vi "svx_DAQ_Facade.vi"(0 "Data In":T13, 2 "Display State In":T2={"Channel Info Array"=[], "Timing Mode"=enum."Time", "Timing Control 1"=25600.0, "Timing Control 2"=2560.0, "Timing Control 3"=16, "Timing Indicator 1"=0.1, "Reference Visible?"=FALSE, "Reference Type"=enum."<none>", "Tachometer Channel"="", "Tach Pulses Per Rev"=1, "Tach Direction"=enum."CW", "Tach Slope"=enum."Rising", "Tach Threshold"=0.0, "Trigger Channel"="", "Trigger Level"=20.0, "Pretrigger Samples"=1, "Trigger Slope"=enum."Falling", "Trigger Hysteresis"=0.0, "Logging Visible?"=FALSE, "Enable Logging"=FALSE, "Logfile Path"=path "c:/test.tdms"} caption="State" {"Timing Control 2" format="%#_6f"; "Channel Info Array"."Max" min=0.0 format="± %^#_4g"; "Channel Info Array"."Channel Type" items=["Voltage (V)"=0, "Charge (C)"=9, "-"=99, "SPL (Pa)"=3, "Force (lbf)"=6, "Force (N)"=1, "Acceleration (g) - IEPE"=2, "Acceleration (g) - Charge"=12, "Acceleration (g) - 4 wire DC Voltage"=22, "Velocity (in/s)"=7, "Velocity (mm/s)"=8, "Prox Probe (mil)"=4, "Prox Probe (mm)"=5]}, 3 "Container State":T12) -> (6 "Data Out":T13, 7 "Display State Out":T2={"Channel Info Array"=[], "Timing Mode"=enum."Time", "Timing Control 1"=25600.0, "Timing Control 2"=2560.0, "Timing Control 3"=16, "Timing Indicator 1"=0.1, "Reference Visible?"=FALSE, "Reference Type"=enum."<none>", "Tachometer Channel"="", "Tach Pulses Per Rev"=1, "Tach Direction"=enum."CW", "Tach Slope"=enum."Rising", "Tach Threshold"=0.0, "Trigger Channel"="", "Trigger Level"=20.0, "Pretrigger Samples"=1, "Trigger Slope"=enum."Falling", "Trigger Hysteresis"=0.0, "Logging Visible?"=FALSE, "Enable Logging"=FALSE, "Logfile Path"=path "c:/test.tdms"} {"Timing Control 2" format="%#_6f"; "Channel Info Array"."Max" min=0.0 format="± %^#_4g"; "Channel Info Array"."Channel Type" items=["Voltage (V)"=0, "Charge (C)"=9, "-"=99, "SPL (Pa)"=3, "Force (lbf)"=6, "Force (N)"=1, "Acceleration (g) - IEPE"=2, "Acceleration (g) - Charge"=12, "Acceleration (g) - 4 wire DC Voltage"=22, "Velocity (in/s)"=7, "Velocity (mm/s)"=8, "Prox Probe (mil)"=4, "Prox Probe (mm)"=5]}, 8 "Action":T1)   [LabVIEW 2017, in "SVX NI-DAQmx AI Configuration XControl.xctl"]
uses:
  <vilib>/addons/Sound and Vibration/svt_DAQmx/Configuration XControl/SVX NI-DAQmx AI Configuration XControl.xctl
  <vilib>/addons/Sound and Vibration/svt_DAQmx/Configuration XControl/Controls/svx_DAQ_ChannelInfo.ctl
  <vilib>/addons/Sound and Vibration/svt_DAQmx/Configuration XControl/Controls/svx_DAQ_ChannelType.ctl
  <vilib>/addons/Sound and Vibration/svt_DAQmx/Configuration XControl/Controls/svx_DAQ_Coupling.ctl
  <vilib>/addons/Sound and Vibration/svt_DAQmx/Configuration XControl/Controls/svx_DAQ_Excitation.ctl
  <vilib>/addons/Sound and Vibration/svt_DAQmx/Configuration XControl/Controls/svx_DAQ_TimingType.ctl
  <vilib>/addons/Sound and Vibration/svt_DAQmx/Configuration XControl/SubVIs/svx_DAQ_Data.ctl
  <vilib>/_xctls/Container State.ctl
  <vilib>/addons/Sound and Vibration/svt_DAQmx/Configuration XControl/SubVIs/svx_DAQ_State.ctl
  <vilib>/addons/Sound and Vibration/svt_DAQmx/Configuration XControl/Controls/svx_DAQ_ReferenceType.ctl
  <vilib>/addons/Sound and Vibration/svt_DAQmx/Configuration XControl/Controls/svx_DAQ_RotationDirection.ctl
  <vilib>/addons/Sound and Vibration/svt_DAQmx/Configuration XControl/Controls/svx_DAQ_Tach_Slope.ctl
  <vilib>/addons/Sound and Vibration/svt_DAQmx/Configuration XControl/Controls/svx_DAQ_Trigger_Slope.ctl
  <vilib>/_xctls/Action.ctl
  <vilib>/addons/Sound and Vibration/svt_DAQmx/Configuration XControl/Controls/svx_DAQ_LoadfromXMLButton.ctl
  <vilib>/addons/Sound and Vibration/svt_DAQmx/Configuration XControl/Controls/svx_DAQ_SavetoXMLButton.ctl
  <vilib>/addons/Sound and Vibration/svt_DAQmx/Configuration XControl/Controls/svx_DAQ_DetailsButton.ctl
  <vilib>/addons/Sound and Vibration/svt_DAQmx/Configuration XControl/Controls/svx_DAQ_ControlRefs.ctl
  <vilib>/_xctls/XControlSupport.lvlib
  <vilib>/Utility/miscctls.llb/LVPointTypeDef.ctl
panel:
  in  "Channel Info Array":T3[](array[typedef]) {"Max" min=0.0 format="± %^#_4g"; "Channel Type" items=["Voltage (V)"=0, "Charge (C)"=9, "-"=99, "SPL (Pa)"=3, "Force (lbf)"=6, "Force (N)"=1, "Acceleration (g) - IEPE"=2, "Acceleration (g) - Charge"=12, "Acceleration (g) - 4 wire DC Voltage"=22, "Velocity (in/s)"=7, "Velocity (mm/s)"=8, "Prox Probe (mil)"=4, "Prox Probe (mm)"=5]}
  in  "Trigger Slope":T11=enum."Rising" caption="Slope"
  in  "Tach Slope":T10 caption="Slope"
  in  "Logfile Path":path=path "c:/test.tdms"
  in  "Enable Logging":bool caption="Enable \nTDMS Logging"
  in  "Trigger Hysteresis":dbl caption="Hysteresis"
  in  "Pretrigger Samples":i32=20 caption="Pretrigger"
  in  "Trigger Level":dbl caption="Level"
  in  "Trigger Channel":string(combo)
  in  "Timing Mode":T7
  in  "Reference Type":T8
  in  "Configuration Error":T14 caption="Caption"
  in  "Save to XML":T15 caption="Caption"
  in  "Load From XML":T16 caption="Caption"
  in  "Error Picture":picture
  in  "Tachometer Channel":string(combo)
  in  "Tach Threshold":dbl caption="Threshold"
  in  "Tach Direction":T9=enum."CCW" caption="Direction"
  in  "Tach Pulses Per Rev":i32=1 caption="Pulses/Rev"
  out "Timing Indicator 1":dbl=0.1 caption="Block Duration (s)" format="%_4g"
  in  "Timing Control 3":i32=16 caption="NOT USED" min=0
  in  "Timing Control 2":dbl=2560.0 caption="Block Size" min=0.0 format="%#_6f"
  in  "Timing Control 1":dbl=25600.0 caption="Min Sample Rate (Hz)" min=0.0
  # "NI-DAQmx Channel"
  # "Channel Type (EU)"
  # "Range"
  # "Sensitivity"
  # "Excitation"
  # "Coupling"
  # "Location"
  # "Orientation"
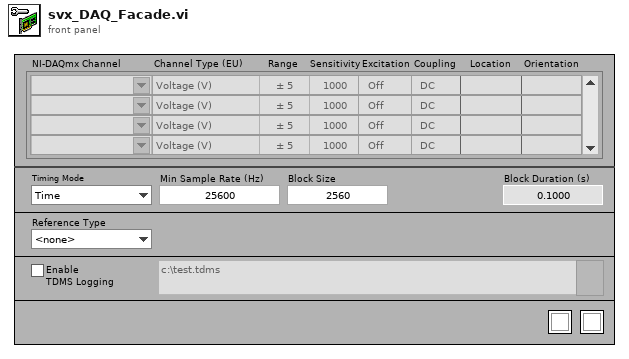
[diagram p1: front panel]
types:
  T1 = typedef "XControlSupport.lvlib/Action.ctl" = cluster{"Data Changed?":bool, "State Changed?":bool, "Action Name":string}
  T2 = typedef "SVX NI-DAQmx AI Configuration XControl.xctl/svx_DAQ_State.ctl" = cluster{"Channel Info Array":T3[], "Timing Mode":T7, "Timing Control 1":dbl, "Timing Control 2":dbl, "Timing Control 3":i32, "Timing Indicator 1":dbl, "Reference Visible?":bool, "Reference Type":T8, "Tachometer Channel":string, "Tach Pulses Per Rev":i32, "Tach Direction":T9, "Tach Slope":T10, "Tach Threshold":dbl, "Trigger Channel":string, "Trigger Level":dbl, "Pretrigger Samples":i32, "Trigger Slope":T11, "Trigger Hysteresis":dbl, "Logging Visible?":bool, "Enable Logging":bool, "Logfile Path":path}
  T3 = typedef "SVX NI-DAQmx AI Configuration XControl.xctl/svx_DAQ_ChannelInfo.ctl" = cluster{"Initialized?":bool, "DAQmx Channel":tag, "Channel Type":T4, "Max":dbl, "Sensitivity":dbl, "Excitation":bool, "Coupling":T5, "Location":string, "Orientation":string, "excitation":T6}
  T4 = typedef "SVX NI-DAQmx AI Configuration XControl.xctl/svx_DAQ_ChannelType.ctl" = u16
  T5 = typedef "SVX NI-DAQmx AI Configuration XControl.xctl/svx_DAQ_Coupling.ctl" = enum16{"AC", "DC"}
  T6 = typedef "svx_DAQ_Excitation.ctl" = enum16{"Off", "Min", "Max"}
  T7 = typedef "SVX NI-DAQmx AI Configuration XControl.xctl/svx_DAQ_TimingType.ctl" = enum16{"Time", "Frequency", "Order"}
  T8 = typedef "SVX NI-DAQmx AI Configuration XControl.xctl/svx_DAQ_ReferenceType.ctl" = enum16{"<none>", "Analog Tachometer", "Analog SW Trigger"}
  T9 = typedef "SVX NI-DAQmx AI Configuration XControl.xctl/svx_DAQ_RotationDirection.ctl" = enum16{"CW", "CCW"}
  T10 = typedef "SVX NI-DAQmx AI Configuration XControl.xctl/svx_DAQ_Tach_Slope.ctl" = enum16{"Rising", "Falling"}
  T11 = typedef "SVX NI-DAQmx AI Configuration XControl.xctl/svx_DAQ_Trigger_Slope.ctl" = enum16{"Falling", "Rising"}
  T12 = typedef "XControlSupport.lvlib/Container State.ctl" = cluster{"Indicator?":bool, "Run Mode?":bool, " Refnum":refnum<vi>}
  T13 = typedef "SVX NI-DAQmx AI Configuration XControl.xctl/svx_DAQ_Data.ctl" = refnum<k21>
  T14 = typedef "SVX NI-DAQmx AI Configuration XControl.xctl/svx_DAQ_DetailsButton.ctl" = bool
  T15 = typedef "SVX NI-DAQmx AI Configuration XControl.xctl/svx_DAQ_SavetoXMLButton.ctl" = bool
  T16 = typedef "SVX NI-DAQmx AI Configuration XControl.xctl/svx_DAQ_LoadfromXMLButton.ctl" = bool
  T17 = typedef "SVX NI-DAQmx AI Configuration XControl.xctl/svx_DAQ_ControlRefs.ctl" = cluster{"Channel Info Array":refnum<vi>, "Timing Mode":refnum<vi>, "Timing Control 1":refnum<vi>, "Timing Control 2":refnum<vi>, "Timing Control 3":refnum<vi>, "Timing Indicator 1":refnum<vi>, "Reference Type":refnum<vi>, "Tachometer Channel":refnum<vi>, "Tach Pulses Per Rev":refnum<vi>, "Tach Direction":refnum<vi>, "Tach Slope":refnum<vi>, "Tach Threshold":refnum<vi>, "Error Picture":refnum<vi>, "Configuration Error":refnum<vi>, "Load From XML":refnum<vi>, "Save to XML":refnum<vi>, "Trigger Channel":refnum<vi>, "Trigger Level":refnum<vi>, "Trigger Slope":refnum<vi>, "Pretrigger Samples":refnum<vi>, "Trigger Hysteresis":refnum<vi>, "Enable Logging":refnum<vi>, "Logfile Path":refnum<vi>, "Task Configuration":refnum<vi>, "Splitter":refnum<vi>}
  T18 = enum8{"Enabled", "Disabled", "Disabled and Grayed Out"}
  T19 = typedef "LVPointTypeDef.ctl" = cluster{"Horizontal":i16, "Vertical":i16}
  T20 = typedef "LVRectTypeDef.ctl" = cluster{"Left":i16, "Top":i16, "Right":i16, "Bottom":i16}
  T21 = typedef "eventvkey.ctl" = enum16{"ASCII", "Enter", "Return", "Shift", "Ctrl", "Alt", "Cmd", "Opt", "Caps", "NumLock", "Clear", "Break", "Up", "Down", "Left", "Right", "Insert", "Delete", "Home", "End", "PageUp", "PageDown", "Escape", "Help", "Pause", "ScrollLock", "F1", "F2", "F3", "F4", "F5", "F6", "F7", "F8", "F9", "F10", "F11", "F12", "F13", "F14", "F15", "F16", "F17", "F18", "F19", "F20", "F21", "F22", "F23", "F24", "Play", "VolumeUp", "VolumeDown", "Mute", "Two Byte Char"}
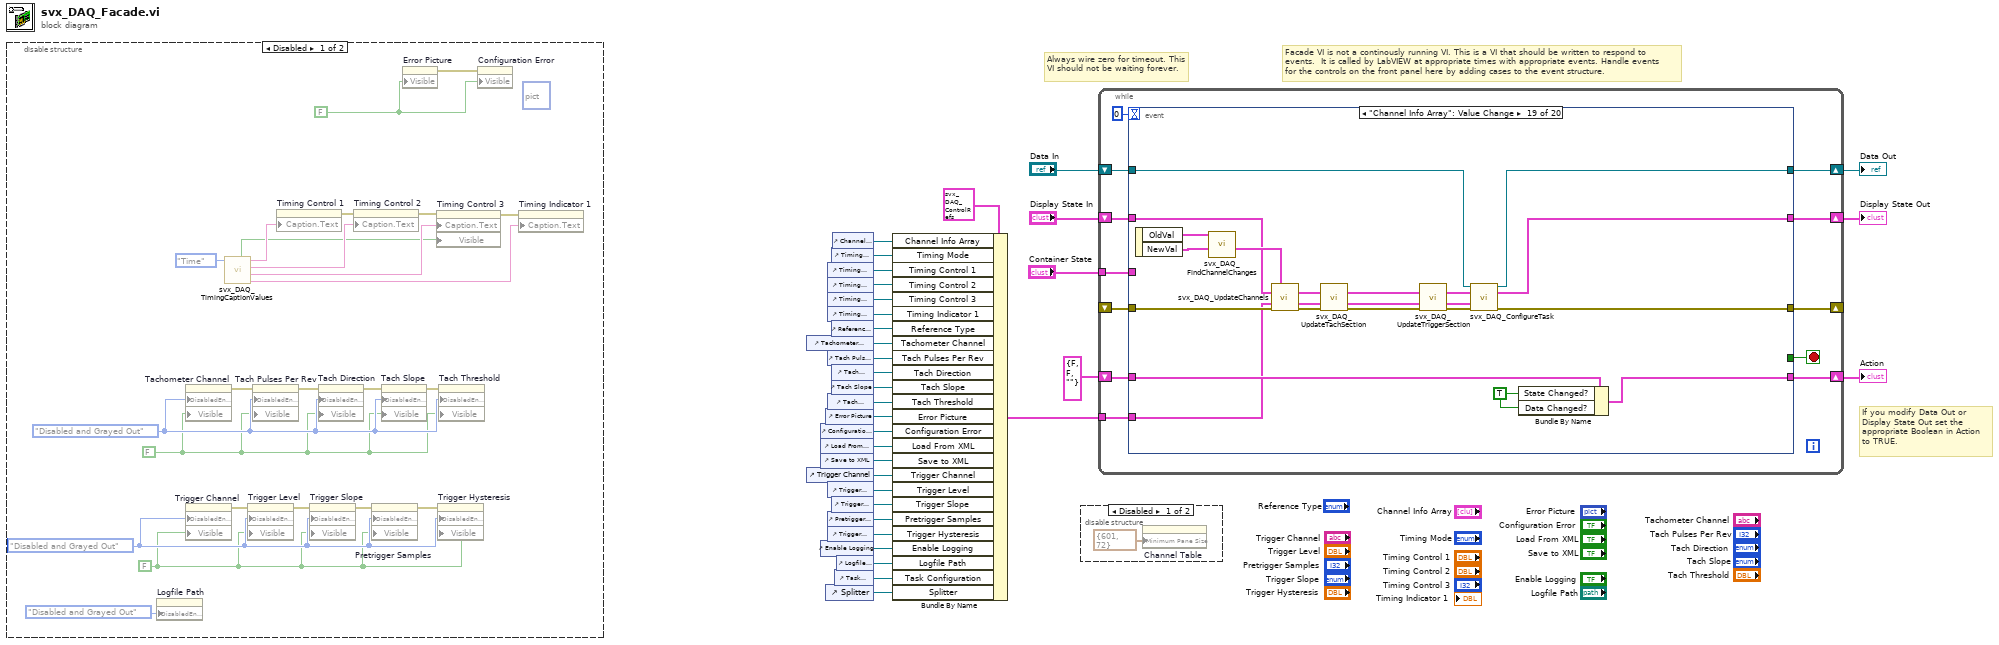
[diagram p0: block diagram]
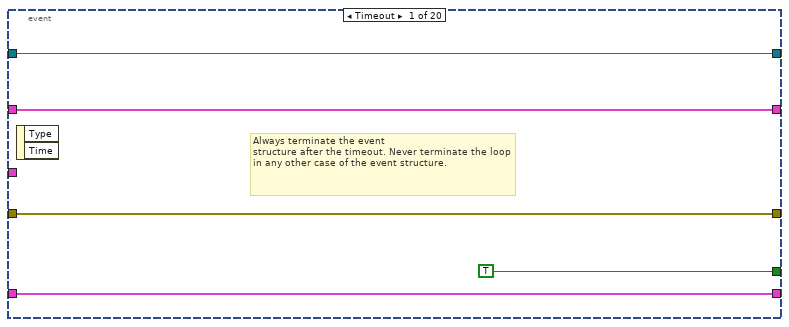
[diagram p4: hidden frame]
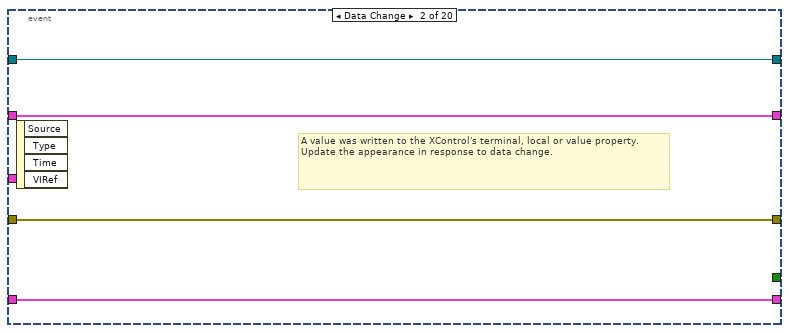
[diagram p5: hidden frame]
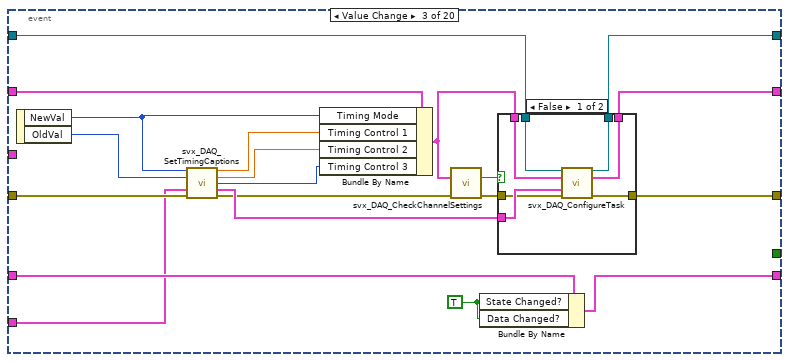
[diagram p6: hidden frame]
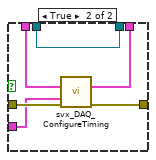
[diagram p7: hidden frame]
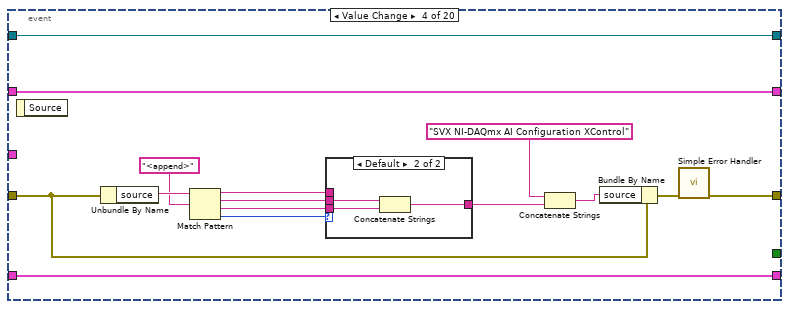
[diagram p8: hidden frame]
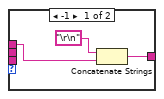
[diagram p9: hidden frame]
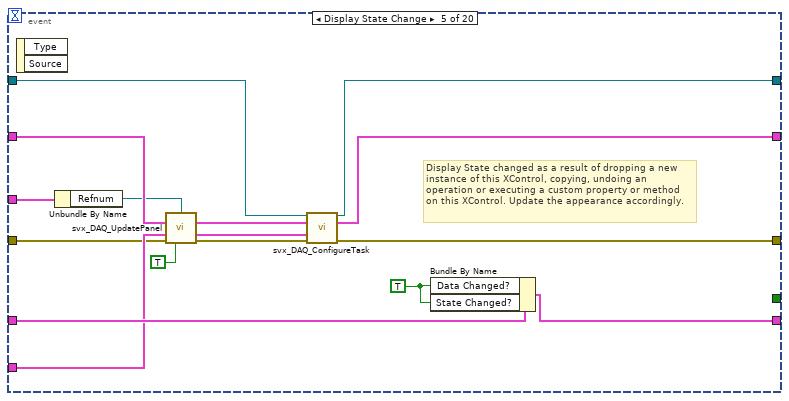
[diagram p10: hidden frame]
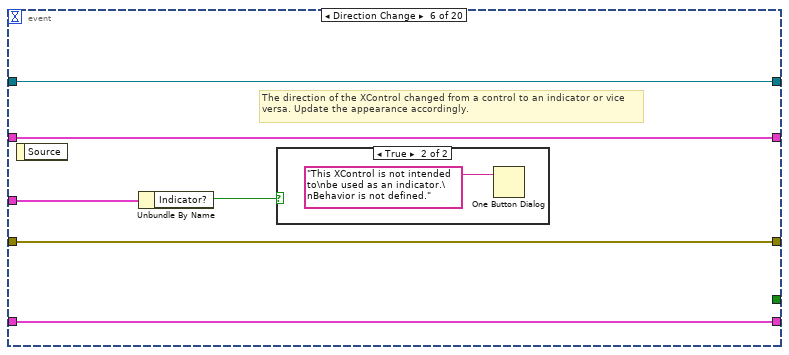
[diagram p11: hidden frame]
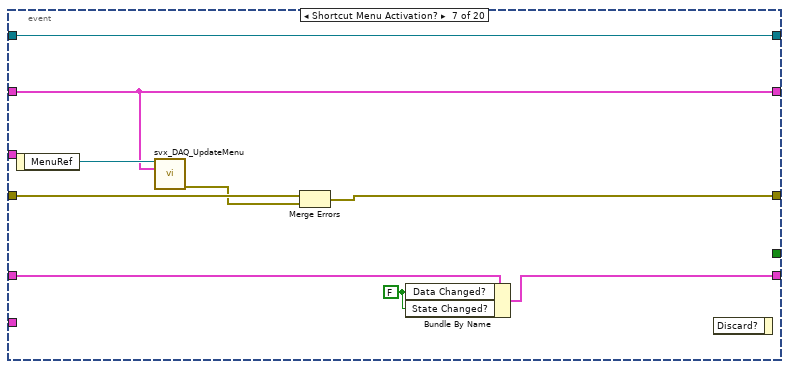
[diagram p13: hidden frame]
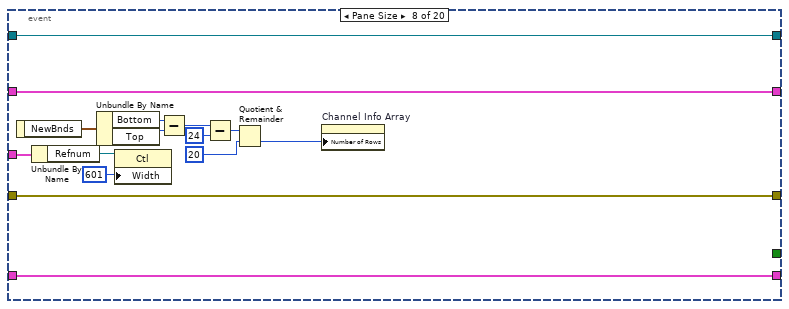
[diagram p14: hidden frame]
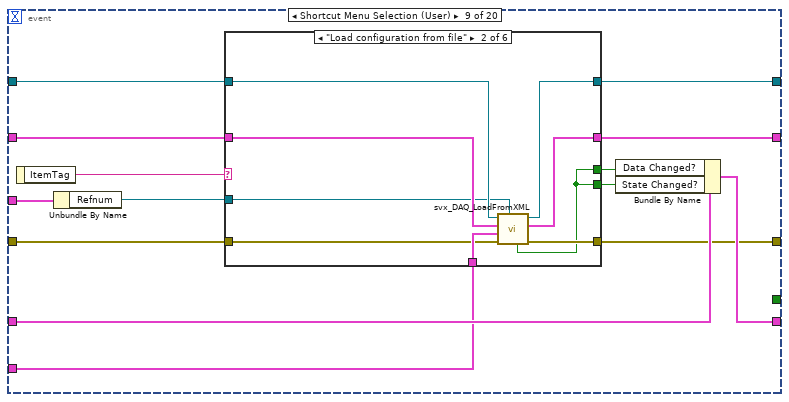
[diagram p15: hidden frame]
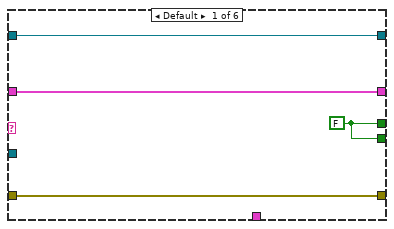
[diagram p16: hidden frame]
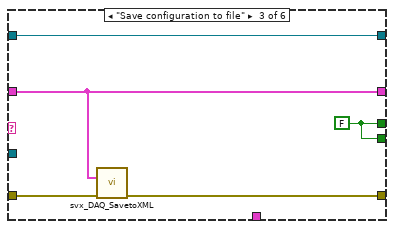
[diagram p17: hidden frame]
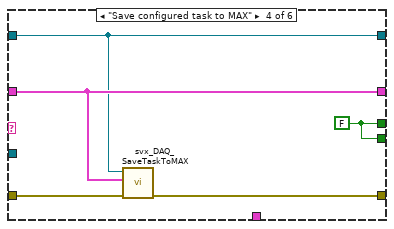
[diagram p18: hidden frame]
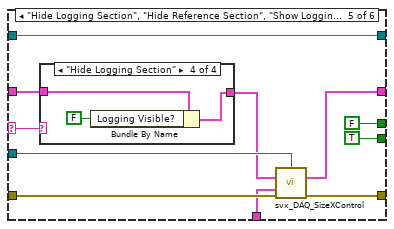
[diagram p19: hidden frame]
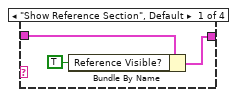
[diagram p20: hidden frame]
diagram:
  # "Facade VI is not a continously running VI. This is a VI that should be written to respond to events.  It is called by LabVIEW at appropriate times with appropriate events. Handle events for the controls on the front panel here by adding cases to the event structure."
  # "Always wire zero for timeout. This\nVI should not be waiting forever."
  # "If you modify Data Out or\nDisplay State Out set the\nappropriate Boolean in Action\nto TRUE."
  n1 = disable-structure shown="Disabled" {
    frame Disabled {
      w38 = FALSE ("Visible")
      w39 = T18."Disabled and Grayed Out" ("Disabled")
      w40 = FALSE ("Visible")
      w41 = T18."Disabled and Grayed Out" ("Disabled")
      (unwired) picture bytes[2913] ("Error Picture")
      w55 = FALSE ("Visible")
      n2 = property on="Logfile Path" class="Path"("DisabledEnum"=T18."Disabled and Grayed Out" ("Disabled")) -> ()  [unwired: 2 in, 2 out]
      n3 = property on="Tachometer Channel" class="CmbBox"("DisabledEnum"=w41, "Visible"=w40) -> (error out=w47:errorcluster)  [unwired: 2 in, 1 out]
      n4 = property on="Trigger Channel" class="CmbBox"("DisabledEnum"=w39, "Visible"=w38) -> (error out=w45:errorcluster)  [unwired: 2 in, 1 out]
      n5 = call <vilib>:"svx_DAQ_TimingCaptionValues.vi"("Timing Mode"=svx_DAQ_TimingType."Time") -> ("Timing Indicator 1 Caption"=w50:string, "Timing Control 3 Caption"=w51:string, "Timing Control 2 Caption"=w57:string, "Timing Control 1 Caption"=w58:string, "Timing Control 3 Visible?"=w49:bool)  [unwired: 6 in]
      n6 = property on="Trigger Level" class="DigNum (strict)"(error in=w45, "DisabledEnum"=w39, "Visible"=w38) -> (error out=w37:errorcluster)  [unwired: 1 in, 1 out]
      n7 = property on="Tach Pulses Per Rev" class="DigNum (strict)"(error in=w47, "DisabledEnum"=w41, "Visible"=w40) -> (error out=w48:errorcluster)  [unwired: 1 in, 1 out]
      n8 = property on="Timing Control 1" class="DigNum (strict)"("Caption.Text"=w58) -> (error out=w56:errorcluster)  [unwired: 2 in, 1 out]
      n9 = property on="Trigger Slope" class="Enum (strict)"(error in=w37, "DisabledEnum"=w39, "Visible"=w38) -> (error out=w36:errorcluster)  [unwired: 1 in, 1 out]
      n10 = property on="Tach Direction" class="Enum (strict)"(error in=w48, "DisabledEnum"=w41, "Visible"=w40) -> (error out=w43:errorcluster)  [unwired: 1 in, 1 out]
      n11 = property on="Timing Control 2" class="DigNum (strict)"(error in=w56, "Caption.Text"=w57) -> (error out=w53:errorcluster)  [unwired: 1 in, 1 out]
      n12 = property on="Pretrigger Samples" class="DigNum (strict)"(error in=w36, "DisabledEnum"=w39, "Visible"=w38) -> (error out=w46:errorcluster)  [unwired: 1 in, 1 out]
      n13 = property on="Tach Slope" class="Enum (strict)"(error in=w43, "DisabledEnum"=w41, "Visible"=w40) -> (error out=w42:errorcluster)  [unwired: 1 in, 1 out]
      n14 = property on="Error Picture" class="Pict"("Visible"=w55) -> (error out=w54:errorcluster)  [unwired: 2 in, 1 out]
      n15 = property on="Timing Control 3" class="DigNum (strict)"(error in=w53, "Caption.Text"=w51, "Visible"=w49) -> (error out=w52:errorcluster)  [unwired: 1 in, 1 out]
      n16 = property on="Trigger Hysteresis" class="DigNum (strict)"(error in=w46, "DisabledEnum"=w39, "Visible"=w38) -> ()  [unwired: 1 in, 2 out]
      n17 = property on="Tach Threshold" class="DigNum (strict)"(error in=w42, "DisabledEnum"=w41, "Visible"=w40) -> ()  [unwired: 1 in, 2 out]
      n18 = property on="Configuration Error" class="Bool"(error in=w54, "Visible"=w55) -> ()  [unwired: 1 in, 2 out]
      n19 = property on="Timing Indicator 1" class="DigNum (strict)"(error in=w52, "Caption.Text"=w50) -> ()  [unwired: 1 in, 2 out]
    }
    frame Enabled {
    }
  }
  n20 = control-ref of="Tachometer Channel"() -> (w24:refnum<vi>)
  n21 = control-ref of="Trigger Channel"() -> (w13:refnum<vi>)
  n22 = control-ref of="Configuration Error"() -> (w19:refnum<vi>)
  n23 = control-ref of="Load From XML"() -> (w18:refnum<vi>)
  n24 = control-ref of="Save to XML"() -> (w17:refnum<vi>)
  n25 = control-ref of="Enable Logging"() -> (w8:refnum<vi>)
  n26 = control-ref of="Error Picture"() -> (w20:refnum<vi>)
  n27 = control-ref of="Splitter"() -> (w3:refnum<vi>)
  n28 = control-ref of="Timing Control 1"() -> (w27:refnum<vi>)
  n29 = control-ref of="Timing Control 2"() -> (w26:refnum<vi>)
  n30 = control-ref of="Timing Control 3"() -> (w16:refnum<vi>)
  n31 = control-ref of="Timing Indicator 1"() -> (w25:refnum<vi>)
  n32 = control-ref of="Tach Pulses Per Rev"() -> (w23:refnum<vi>)
  n33 = control-ref of="Tach Threshold"() -> (w21:refnum<vi>)
  n34 = control-ref of="Trigger Level"() -> (w12:refnum<vi>)
  n35 = control-ref of="Pretrigger Samples"() -> (w11:refnum<vi>)
  n36 = control-ref of="Trigger Hysteresis"() -> (w10:refnum<vi>)
  n37 = control-ref of="Timing Mode"() -> (w14:refnum<vi>)
  n38 = control-ref of="Reference Type"() -> (w9:refnum<vi>)
  n39 = control-ref of="Tach Direction"() -> (w22:refnum<vi>)
  n40 = control-ref of="Tach Slope"() -> (w6:refnum<vi>)
  n41 = control-ref of="Trigger Slope"() -> (w5:refnum<vi>)
  n42 = control-ref of="Channel Info Array"() -> (w1:refnum<vi>)
  n43 = control-ref of="Task Configuration"() -> (w4:refnum<vi>)
  n44 = control-ref of="Logfile Path"() -> (w7:refnum<vi>)
  n45 = Bundle By Name(cluster=T17 {"Channel Info Array"=refnum, "Timing Mode"=refnum, "Timing Control 1"=refnum, "Timing Control 2"=refnum, "Timing Control 3"=refnum, "Timing Indicator 1"=refnum, "Reference Type"=refnum, "Tachometer Channel"=refnum, "Tach Pulses Per Rev"=refnum, "Tach Direction"=refnum, "Tach Slope"=refnum, "Tach Threshold"=refnum, "Error Picture"=refnum, "Configuration Error"=refnum, "Load From XML"=refnum, "Save to XML"=refnum, "Trigger Channel"=refnum, "Trigger Level"=refnum, "Trigger Slope"=refnum, "Pretrigger Samples"=refnum, "Trigger Hysteresis"=refnum, "Enable Logging"=refnum, "Logfile Path"=refnum, "Task Configuration"=refnum, "Splitter"=refnum}, "Channel Info Array"=w1, "Timing Mode"=w14, "Timing Control 1"=w27, "Timing Control 2"=w26, "Timing Control 3"=w16, "Timing Indicator 1"=w25, "Reference Type"=w9, "Tachometer Channel"=w24, "Tach Pulses Per Rev"=w23, "Tach Direction"=w22, "Tach Slope"=w6, "Tach Threshold"=w21, "Error Picture"=w20, "Configuration Error"=w19, "Load From XML"=w18, "Save to XML"=w17, "Trigger Channel"=w13, "Trigger Level"=w12, "Trigger Slope"=w5, "Pretrigger Samples"=w11, "Trigger Hysteresis"=w10, "Enable Logging"=w8, "Logfile Path"=w7, "Task Configuration"=w4, "Splitter"=w3) -> (w29:T17)
  n46 = disable-structure shown="Disabled" {
    frame Disabled {
      n47 = property on="Channel Table" class="Pane"("Minimum Pane Size"=T19 {"Horizontal"=601, "Vertical"=72}) -> ()  [unwired: 2 in, 2 out]
    }
    frame Enabled {
    }
  }
  n48 = while {
    shift-right: [w70] -> w32
    shift-left: "Display State In" -> [w71]
    tunnel: "Container State" -> [w67]
    shift-right: [w60] -> w28
    shift-left: "Data In" -> [w66]
    shift-right: [w64] -> w31
    shift-left: T1 {"Data Changed?"=FALSE, "State Changed?"=FALSE, "Action Name"=""} ("Action") -> [w65]
    tunnel: w29 -> [w63]
    shift-right: [w62] -> _
    shift-left: _ -> [w61]
    stop <- w69 stop-if-true
    n49 = event shown="[18] \"Channel Info Array\": Value Change" {
      selector: _ -> [_ _ _ _ _ _ _ _ _ _ _ _ _ _ _ _ _ _ _ _]
      dyn-events: _ -> [_ _ _ _ _ _ _ _ _ _ _ _ _ _ _ _ _ _ _ _]
      timeout: 0 -> [_ _ _ _ _ _ _ _ _ _ _ _ _ _ _ _ _ _ _ _]
      tunnel: w71 -> [w74 w79 w97 w128 w143 w155 w164 w180 w195 w268 w301 w309 w316 w334 w360 w398 w440 w461 w510 w530]
      tunnel: [w74 w79 w92 w128 w145 w155 w164 w180 w188 w267 w291 w310 w316 w331 w357 w402 w443 w458 w511 w530] -> w70
      tunnel: [TRUE _ _ _ _ _ _ _ _ _ _ _ _ _ _ _ _ _ _ _] -> w69
      tunnel: w67 -> [_ _ _ _ w137 w156 _ w169 w184 w272 _ w305 _ _ _ _ _ _ _ _]
      tunnel: w66 -> [w72 w78 w85 w126 w150 w153 w166 w181 w187 w266 w293 w311 w317 w330 w359 w404 w445 w460 w513 w535]
      tunnel: [w72 w78 w96 w126 w149 w153 w166 w181 w189 w263 w292 w313 w317 w329 w358 w403 w444 w459 w518 w535] -> w60
      tunnel: [w75 w80 w99 w127 w147 w154 w161 w178 w193 w264 w299 w302 w318 w335 w361 w405 w446 w463 w520 w529] -> w64
      tunnel: w65 -> [w75 w80 w100 w127 w148 w154 w163 w178 w194 w265 w300 w303 w318 w336 w362 w406 w447 w464 w519 w529]
      tunnel: w63 -> [_ _ w91 _ w142 _ _ _ w186 w269 w296 w312 _ w321 w353 w395 w438 w453 w515 _]
      tunnel: [w73 w77 w94 w125 w144 w152 w158 w179 w190 w270 w295 w308 w314 w332 w356 w401 w442 w457 w512 w532] -> w62
      tunnel: w61 -> [w73 w77 w93 w121 w141 w152 w160 w179 w192 w271 w297 w307 w315 w325 w355 w396 w436 w454 w516 w532]
      event Timeout {
        # "Always terminate the event\nstructure after the timeout. Never terminate the loop in any other case of the event structure."
        n50 = event-data() -> ()  [unwired: 1 in, 2 out]
      }
      event Data Change {
        # "A value was written to the XControl's terminal, local or value property.\nUpdate the appearance in response to data change."
        n51 = event-data() -> ()  [unwired: 1 in, 4 out]
      }
      event Value Change {
        w95 = TRUE ("State Changed?")
        n52 = event-data() -> ("NewVal"=w98:T7, "OldVal"=w89:T7)  [unwired: 1 in]
        n53 = call <vilib>:"svx_DAQ_SetTimingCaptions.vi"("Timing Mode (new)"=w98, "Timing Mode (old)"=w89, "Reference Cluster"=w91, "error in (no error)"=w93) -> ("Timing Control 1"=w88:dbl, "Timing Control 2"=w87:dbl, "Timing Control 3"=w86:i32, "Reference Cluster Out"=w90:T17, "error out"=w83:errorcluster)  [unwired: 7 in]
        n54 = Bundle By Name(cluster=w97, "Timing Mode"=w98, "Timing Control 1"=w88, "Timing Control 2"=w87, "Timing Control 3"=w86) -> (w84:T2)
        n55 = call <vilib>:"svx_DAQ_CheckChannelSettings.vi"("Display State In"=w84, "error in (no error)"=w83) -> ("Empty Channel List?"=w81:bool, "error out"=w82:errorcluster)  [unwired: 9 in, 3 out]
        n56 = Bundle By Name(cluster=w100, "State Changed?"=w95, "Data Changed?"=w95) -> (w99:T1)
        n57 = case shown="False" w81 {
          tunnel: [w107 w108] -> w96
          tunnel: [w106 w112] -> w94
          tunnel: [w105 w110] -> w92
          tunnel: w90 -> [w104 w109]
          tunnel: w85 -> [w103 w108]
          tunnel: w84 -> [w102 w111]
          tunnel: w82 -> [w101 w113]
          frame False {
            n58 = call <vilib>:"svx_DAQ_ConfigureTask.vi"("Task In"=w103, "Display State In"=w102, "cluster"=w104, "error in"=w101) -> ("task out"=w107:refnum<k21>, "Display State Out"=w105:T2, "error out"=w106:errorcluster)  [unwired: 8 in, 1 out]
          }
          frame True {
            n59 = call <vilib>:"svx_DAQ_ConfigureTiming.vi"("Display State In"=w111, "cluster"=w109, "Error In (no error)"=w113) -> ("Display State Out"=w110:T2, "error out"=w112:errorcluster)  [unwired: 9 in, 2 out]
          }
        }
      }
      event Value Change {
        n60 = event-data() -> ()  [unwired: 1 in, 1 out]
        n61 = Unbundle By Name(w121) -> ("source"=w124:string)
        n62 = Match Pattern(string=w124, regular expression="<append>") -> (before substring=w117:string, match substring=w116:string, after substring=w115:string, offset past match=w119:i32)  [unwired: 1 in]
        n63 = case shown="Default" w119 {
          tunnel: [w129 w132] -> w118
          tunnel: w117 -> [w130 _]
          tunnel: w116 -> [_ w134]
          tunnel: w115 -> [_ w133]
          frame -1 {
            n64 = Concatenate Strings("\r\n", w130) -> (w129:string)
          }
          frame Default {
            n65 = Concatenate Strings(w134, w133) -> (w132:string)
          }
        }
        n66 = Concatenate Strings("SVX NI-DAQmx AI Configuration XControl" ("error source (\" \")"), w118) -> (w114:string)
        n67 = Bundle By Name(cluster=w121, "source"=w114) -> (w120:errorcluster)
        n68 = call <vilib>:"Simple Error Handler.vi"("error in (no error)"=w120) -> ("error out"=w125:errorcluster)  [unwired: 4 in, 4 out]
      }
      event Display State Change {
        w146 = TRUE ("Data Changed?")
        # "Display State changed as a result of dropping a new instance of this XControl, copying, undoing an operation or executing a custom property or method on this XControl. Update the appearance accordingly."
        n69 = event-data() -> ()  [unwired: 1 in, 2 out]
        n70 = Unbundle By Name(w137) -> ("Refnum"=w136:refnum<vi>)
        n71 = call <vilib>:"svx_DAQ_UpdatePanel.vi"("XControl Ref"=w136, "State"=w143, "cluster"=w142, "error in (no error)"=w141, "display state change"=TRUE) -> ("State Out"=w138:T2, "cluster"=w139:T17, "error out"=w140:errorcluster)  [unwired: 8 in]
        n72 = call <vilib>:"svx_DAQ_ConfigureTask.vi"("Task In"=w150, "Display State In"=w138, "cluster"=w139, "error in"=w140) -> ("task out"=w149:refnum<k21>, "Display State Out"=w145:T2, "error out"=w144:errorcluster)  [unwired: 8 in, 1 out]
        n73 = Bundle By Name(cluster=w148, "Data Changed?"=w146, "State Changed?"=w146) -> (w147:T1)
      }
      event Direction Change {
        # "The direction of the XControl changed from a control to an indicator or vice versa. Update the appearance accordingly."
        n74 = event-data() -> ()  [unwired: 1 in, 1 out]
        n75 = Unbundle By Name(w156) -> ("Indicator?"=w151:bool)
        n76 = case shown="True" w151 {
          frame False {
          }
          frame True {
            n77 = One Button Dialog(message="This XControl is not intended to\nbe used as an indicator.\nBehavior is not defined.") -> ()  [unwired: 1 in, 1 out]
          }
        }
      }
      event Shortcut Menu Activation? {
        w162 = FALSE ("Data Changed?")
        n78 = event-data() -> ("MenuRef"=w165:refnum<k9>)  [unwired: 1 in]
        n79 = call <vilib>:"svx_DAQ_UpdateMenu.vi"("MenuRef"=w165, "Display State In"=w164) -> ("error out"=w159:errorcluster)  [unwired: 13 in]
        n80 = Merge Errors(w160, w159) -> (w158:errorcluster)
        n81 = Bundle By Name(cluster=w163, "Data Changed?"=w162, "State Changed?"=w162) -> (w161:T1)
        n82 = event-data() -> ()  [unwired: 2 in, 1 out]
      }
      event Pane Size {
        n83 = event-data() -> ("NewBnds"=w177:T20)  [unwired: 1 in]
        n84 = Unbundle By Name(w169) -> ("Refnum"=w168:refnum<vi>)
        n85 = Unbundle By Name(w177) -> ("Bottom"=w175:i16, "Top"=w176:i16)
        n86 = property class="Ctl"(reference=w168, "Width"=u32 601 ("XControl:Container Bounds:Width")) -> ()  [unwired: 1 in, 2 out]
        n87 = Subtract(x=w175, y=w176) -> (x-y=w174:i16)
        n88 = Subtract(x=w174, y=i16 24) -> (x-y=w172:i16)
        n89 = Quotient & Remainder(x=w172, y=i16 20) -> (floor(x/y)=w170:i16)  [unwired: 1 out]
        n90 = property on="Channel Info Array" class="Arr (strict)"("Number of Rows"=w170) -> ()  [unwired: 2 in, 2 out]
      }
      event Shortcut Menu Selection (User) {
        n91 = event-data() -> ("ItemTag"=w191:string)  [unwired: 1 in]
        n92 = Unbundle By Name(w184) -> ("Refnum"=w183:refnum<vi>)
        n93 = case shown="\"Load configuration from file\"" w191 {
          selector: w191 -> [_ _ _ _ w219 _]
          tunnel: w195 -> [w199 w205 w212 w216 w221 w251]
          tunnel: [w199 w206 w212 w216 w223 w244] -> w188
          tunnel: w192 -> [w198 w202 w211 w218 w226 w247]
          tunnel: [w198 w203 w210 w217 w222 w249] -> w190
          tunnel: [w197 w207 w213 w215 w227 w252] -> w189
          tunnel: w187 -> [w197 w208 w213 w215 w227 w252]
          tunnel: w186 -> [_ w204 _ _ w225 w243]
          tunnel: [w196 w201 w209 w214 FALSE ("State and Data Changed?") FALSE ("State and Data Changed?")] -> w185
          tunnel: w183 -> [_ w200 _ _ w224 w248]
          tunnel: [w196 w201 w209 w214 TRUE ("State and Data Changed?") w242] -> w182
          frame Default {
            w196 = FALSE ("State and Data Changed?")
          }
          frame "Load configuration from file" {
            n94 = call <vilib>:"svx_DAQ_LoadFromXML.vi"("XControl Ref"=w200, "error in (no error)"=w202, "cluster"=w204, "Display State In"=w205, "Data In"=w208) -> ("error out"=w203:errorcluster, "Display State Out"=w206:T2, "Data Out"=w207:T13, "State and Data Changed?"=w201:bool)  [unwired: 3 in]
          }
          frame "Save configuration to file" {
            w209 = FALSE ("State and Data Changed?")
            n95 = call <vilib>:"svx_DAQ_SavetoXML.vi"("State"=w212, "error in (no error)"=w211) -> ("error out"=w210:errorcluster)  [unwired: 12 in, 1 out]
          }
          frame "Save configured task to MAX" {
            w214 = FALSE ("State and Data Changed?")
            n96 = call <vilib>:"svx_DAQ_SaveTaskToMAX.vi"("error in (no error)"=w218, "Display State In"=w216, "Task In"=w215) -> ("error out"=w217:errorcluster)  [unwired: 8 in]
          }
          frame "Hide Logging Section", "Hide Reference Section", "Show Logging Section", "Show Reference Section" {
            n97 = case shown="\"Hide Logging Section\"" w219 {
              tunnel: w221 -> [w231 w234 w237 w240]
              tunnel: [w230 w233 w236 w239] -> w220
              frame "Show Reference Section", Default {
                n98 = Bundle By Name(cluster=w231, "Reference Visible?"=TRUE) -> (w230:T2)
              }
              frame "Hide Reference Section" {
                n99 = Bundle By Name(cluster=w234, "Reference Visible?"=FALSE) -> (w233:T2)
              }
              frame "Show Logging Section" {
                n100 = Bundle By Name(cluster=w237, "Logging Visible?"=TRUE ("Reference Visible?")) -> (w236:T2)
              }
              frame "Hide Logging Section" {
                n101 = Bundle By Name(cluster=w240, "Logging Visible?"=FALSE ("Reference Visible?")) -> (w239:T2)
              }
            }
            n102 = call <vilib>:"svx_DAQ_SizeXControl.vi"("XControl Ref"=w224, "State"=w220, "Reference Cluster"=w225, "error in (no error)"=w226) -> ("State Out"=w223:T2, "error out"=w222:errorcluster)  [unwired: 9 in, 1 out]
          }
          frame "Unflatten Channel List" {
            n103 = call <vilib>:"svx_DAQ_ExplodeChannels.vi"("Display State In"=w251, "error in (no error)"=w247) -> ("Display State Out"=w245:T2, "State Updated?"=w242:bool, "error out"=w246:errorcluster)  [unwired: 11 in]
            n104 = case shown="True" w242 {
              tunnel: [w253 w260] -> w249
              tunnel: w248 -> [_ w259]
              tunnel: w246 -> [w253 w258]
              tunnel: w245 -> [w254 w257]
              tunnel: [w254 w256] -> w244
              tunnel: w243 -> [_ w255]
              frame False {
              }
              frame True {
                n105 = call <vilib>:"svx_DAQ_UpdatePanel.vi"("XControl Ref"=w259, "State"=w257, "cluster"=w255, "error in (no error)"=w258) -> ("State Out"=w256:T2, "error out"=w260:errorcluster)  [unwired: 9 in, 1 out]
              }
            }
          }
        }
        n106 = Bundle By Name(cluster=w194, "Data Changed?"=w185, "State Changed?"=w182) -> (w193:T1)
      }
      event Exec State Change {
        # "The VI owning the XControl changed from Edit Mode  to Run Mode or vice versa.\nUpdate the appearance accordingly."
        # "Handle Edit Mode & Run Mode\ncase differently"
        n107 = event-data() -> ()  [unwired: 1 in, 1 out]
        n108 = Unbundle By Name(w272) -> ("Run Mode?"=w261:bool)
        n109 = case shown="False" w261 {
          tunnel: w271 -> [w279 w280]
          tunnel: [w278 w280] -> w270
          tunnel: w269 -> [w277 _]
          tunnel: w268 -> [w276 w282]
          tunnel: [w275 w282] -> w267
          tunnel: [w274 w281] -> w263
          tunnel: w266 -> [w273 w281]
          frame False {
            n110 = call <vilib>:"svx_DAQ_ConfigureTask.vi"("Task In"=w273, "Display State In"=w276, "cluster"=w277, "error in"=w279) -> ("task out"=w274:refnum<k21>, "Display State Out"=w275:T2, "error out"=w278:errorcluster)  [unwired: 8 in, 1 out]
          }
          frame True {
          }
        }
        n111 = Not(x=w261) -> (.not. x?=w262:bool)
        n112 = Bundle By Name(cluster=w265, "Data Changed?"=w262) -> (w264:T1)
      }
      event Value Change {
        n113 = event-data() -> ("NewVal"=w289:T8)  [unwired: 1 in]
        n114 = Bundle By Name(cluster=w301, "Reference Type"=w289) -> (w290:T2)
        n115 = call <vilib>:"svx_DAQ_UpdateTachSection.vi"("State"=w290, "cluster"=w296, "error in (no error)"=w297) -> ("State Out"=w284:T2, "cluster"=w286:T17, "error out"=w288:errorcluster)  [unwired: 10 in]
        n116 = call <vilib>:"svx_DAQ_UpdateTriggerSection.vi"("State"=w284, "Reference Cluster"=w286, "error in (no error)"=w288) -> ("State Out"=w283:T2, "Reference Cluster Out"=w285:T17, "error out"=w287:errorcluster)  [unwired: 10 in]
        n117 = call <vilib>:"svx_DAQ_ConfigureTask.vi"("Task In"=w293, "Display State In"=w283, "cluster"=w285, "error in"=w287) -> ("task out"=w292:refnum<k21>, "Display State Out"=w291:T2, "error out"=w295:errorcluster)  [unwired: 8 in, 1 out]
        n118 = Bundle By Name(cluster=w300, "State Changed?"=TRUE, "Data Changed?"=TRUE ("State Changed?")) -> (w299:T1)
      }
      event Value Change {
        n119 = event-data() -> ()  [unwired: 1 in, 1 out]
        n120 = Unbundle By Name(w305) -> ("Refnum"=w304:refnum<vi>)
        n121 = call <vilib>:"svx_DAQ_LoadFromXML.vi"("XControl Ref"=w304, "error in (no error)"=w307, "cluster"=w312, "Display State In"=w309, "Data In"=w311) -> ("error out"=w308:errorcluster, "Display State Out"=w310:T2, "Data Out"=w313:T13, "State and Data Changed?"=w306:bool)  [unwired: 3 in]
        n122 = Bundle By Name(cluster=w303, "State Changed?"=w306, "Data Changed?"=w306) -> (w302:T1)
      }
      event Value Change {
        n123 = event-data() -> ()  [unwired: 1 in, 1 out]
        n124 = call <vilib>:"svx_DAQ_SavetoXML.vi"("State"=w316, "error in (no error)"=w315) -> ("error out"=w314:errorcluster)  [unwired: 12 in, 1 out]
      }
      event "Enable Logging": Value Change {
        n125 = event-data() -> ("NewVal"=w333:bool)  [unwired: 1 in]
        n126 = Bundle By Name(cluster=w334, "Enable Logging"=w333) -> (w323:T2)
        n127 = call <vilib>:"svx_DAQ_UpdateLogSection.vi"("State"=w323, "Reference Cluster"=w321, "error in (no error)"=w325) -> ("State Out"=w322:T2, "error out"=w324:errorcluster)  [unwired: 10 in, 1 out]
        n128 = call <vilib>:"svx_DAQ_CheckChannelSettings.vi"("Display State In"=w322, "error in (no error)"=w324) -> ("Empty Channel List?"=w320:bool, "error out"=w328:errorcluster)  [unwired: 9 in, 3 out]
        n129 = Not(x=w320) -> (.not. x?=w319:bool)
        n130 = case shown="True" w319 {
          tunnel: [w338 w348] -> w332
          tunnel: w321 -> [_ w347]
          tunnel: [w339 w346] -> w331
          tunnel: w330 -> [w340 w345]
          tunnel: [w340 w344] -> w329
          tunnel: w328 -> [w338 w343]
          tunnel: w323 -> [w339 w342]
          tunnel: [FALSE ("Data Changed?") TRUE ("Data Changed?")] -> w327
          frame False {
          }
          frame True {
            n131 = call <vilib>:"svx_DAQ_ConfigureTask.vi"("Task In"=w345, "Display State In"=w342, "cluster"=w347, "error in"=w343) -> ("task out"=w344:refnum<k21>, "Display State Out"=w346:T2, "error out"=w348:errorcluster)  [unwired: 8 in, 1 out]
          }
        }
        n132 = Bundle By Name(cluster=w336, "Data Changed?"=w327, "State Changed?"=TRUE) -> (w335:T1)
      }
      event "Tach Pulses Per Rev", "Tach Threshold", "Tachometer Channel": Value Change {
        w349 = TRUE ("State Changed?")
        n133 = event-data() -> ("NewVal"=w363:variant, "CtlRef"=w365:refnum<vi>)  [unwired: 1 in]
        n134 = property class="Ctl"(reference=w365) -> ("Label.Text"=w364:string)  [unwired: 1 in, 2 out]
        n135 = case shown="\"Tachometer Channel\", Default" w364 {
          tunnel: w363 -> [w370 w375 w380 w385 w390]
          tunnel: w360 -> [w369 w374 w379 w384 w389]
          tunnel: [w368 w373 w378 w383 w388] -> w351
          frame "Tachometer Channel", Default {
            n136 = Variant To Data(type="" ("Tachometer Channel"), Variant=w370) -> (data=w366:string)  [unwired: 1 in, 1 out]
            n137 = Bundle By Name(cluster=w369, "Tachometer Channel"=w366) -> (w368:T2)
          }
          frame "Tach Pulses Per Rev" {
            n138 = Variant To Data(type=0 ("Pulses Per Rev"), Variant=w375) -> (data=w372:i32)  [unwired: 1 in, 1 out]
            n139 = Bundle By Name(cluster=w374, "Tach Pulses Per Rev"=w372) -> (w373:T2)
          }
          frame "Tach Direction" {
            n140 = Variant To Data(type=svx_DAQ_RotationDirection."CCW" ("Direction"), Variant=w380) -> (data=w377:T9)  [unwired: 1 in, 1 out]
            n141 = Bundle By Name(cluster=w379, "Tach Direction"=w377) -> (w378:T2)
          }
          frame "Tach Slope" {
            n142 = Variant To Data(type=svx_DAQ_Tach_Slope."Rising" ("Tach Slope"), Variant=w385) -> (data=w382:T10)  [unwired: 1 in, 1 out]
            n143 = Bundle By Name(cluster=w384, "Tach Slope"=w382) -> (w383:T2)
          }
          frame "Tach Threshold" {
            n144 = Variant To Data(type=0.0 ("Threshold"), Variant=w390) -> (data=w387:dbl)  [unwired: 1 in, 1 out]
            n145 = Bundle By Name(cluster=w389, "Tach Threshold"=w387) -> (w388:T2)
          }
        }
        n146 = call <vilib>:"svx_DAQ_UpdateTachSection.vi"("State"=w351, "cluster"=w353, "error in (no error)"=w355) -> ("State Out"=w350:T2, "cluster"=w352:T17, "error out"=w354:errorcluster)  [unwired: 10 in]
        n147 = Bundle By Name(cluster=w362, "Data Changed?"=w349, "State Changed?"=w349) -> (w361:T1)
        n148 = call <vilib>:"svx_DAQ_ConfigureTask.vi"("Task In"=w359, "Display State In"=w350, "cluster"=w352, "error in"=w354) -> ("task out"=w358:refnum<k21>, "Display State Out"=w357:T2, "error out"=w356:errorcluster)  [unwired: 8 in, 1 out]
      }
      event "Trigger Channel", "Trigger Level", "Pretrigger Samples", "Trigger Hysteresis": Value Change {
        w400 = TRUE ("State Changed?")
        n149 = event-data() -> ("NewVal"=w397:variant, "CtlRef"=w407:refnum<vi>)  [unwired: 1 in]
        n150 = property class="Ctl"(reference=w407) -> ("Label.Text"=w399:string)  [unwired: 1 in, 2 out]
        n151 = case shown="\"Trigger Hysteresis\"" w399 {
          tunnel: w397 -> [w412 w417 w422 w427 w432]
          tunnel: w398 -> [w411 w416 w421 w426 w431]
          tunnel: [w410 w415 w420 w425 w430] -> w391
          frame "Trigger Channel", Default {
            n152 = Variant To Data(type="" ("Trigger Channel"), Variant=w412) -> (data=w409:string)  [unwired: 1 in, 1 out]
            n153 = Bundle By Name(cluster=w411, "Trigger Channel"=w409) -> (w410:T2)
          }
          frame "Trigger Level" {
            n154 = Variant To Data(type=0.0 ("Trigger Level"), Variant=w417) -> (data=w414:dbl)  [unwired: 1 in, 1 out]
            n155 = Bundle By Name(cluster=w416, "Trigger Level"=w414) -> (w415:T2)
          }
          frame "Pretrigger Samples" {
            n156 = Variant To Data(type=0 ("Pretrigger Samples"), Variant=w422) -> (data=w419:i32)  [unwired: 1 in, 1 out]
            n157 = Bundle By Name(cluster=w421, "Pretrigger Samples"=w419) -> (w420:T2)
          }
          frame "Trigger Slope" {
            n158 = Variant To Data(type=svx_DAQ_Trigger_Slope."Rising" ("Trigger Slope"), Variant=w427) -> (data=w423:T11)  [unwired: 1 in, 1 out]
            n159 = Bundle By Name(cluster=w426, "Trigger Slope"=w423) -> (w425:T2)
          }
          frame "Trigger Hysteresis" {
            n160 = Variant To Data(type=0.0 ("Trigger Hysteresis"), Variant=w432) -> (data=w429:dbl)  [unwired: 1 in, 1 out]
            n161 = Bundle By Name(cluster=w431, "Trigger Hysteresis"=w429) -> (w430:T2)
          }
        }
        n162 = call <vilib>:"svx_DAQ_UpdateTriggerSection.vi"("State"=w391, "Reference Cluster"=w395, "error in (no error)"=w396) -> ("State Out"=w392:T2, "Reference Cluster Out"=w393:T17, "error out"=w394:errorcluster)  [unwired: 10 in]
        n163 = Bundle By Name(cluster=w406, "Data Changed?"=w400, "State Changed?"=w400) -> (w405:T1)
        n164 = call <vilib>:"svx_DAQ_ConfigureTask.vi"("Task In"=w404, "Display State In"=w392, "cluster"=w393, "error in"=w394) -> ("task out"=w403:refnum<k21>, "Display State Out"=w402:T2, "error out"=w401:errorcluster)  [unwired: 8 in, 1 out]
      }
      event "Logfile Path": Value Change {
        w441 = TRUE ("State Changed?")
        n165 = event-data() -> ("NewVal"=w439:path)  [unwired: 1 in]
        n166 = Bundle By Name(cluster=w440, "Logfile Path"=w439) -> (w437:T2)
        n167 = call <vilib>:"svx_DAQ_UpdateLogSection.vi"("State"=w437, "Reference Cluster"=w438, "error in (no error)"=w436) -> ("State Out"=w433:T2, "Reference Cluster Out"=w434:T17, "error out"=w435:errorcluster)  [unwired: 10 in]
        n168 = Bundle By Name(cluster=w447, "Data Changed?"=w441, "State Changed?"=w441) -> (w446:T1)
        n169 = call <vilib>:"svx_DAQ_ConfigureTask.vi"("Task In"=w445, "Display State In"=w433, "cluster"=w434, "error in"=w435) -> ("task out"=w444:refnum<k21>, "Display State Out"=w443:T2, "error out"=w442:errorcluster)  [unwired: 8 in, 1 out]
      }
      event "Timing Control 1", "Timing Control 2", "Timing Control 3": Value Change {
        n170 = event-data() -> ("NewVal"=w465:variant, "CtlRef"=w467:refnum<vi>)  [unwired: 1 in]
        n171 = property class="DigNum"(reference=w467) -> ("Label.Text"=w466:string)  [unwired: 1 in, 2 out]
        n172 = case shown="\"Timing Control 1\"" w466 {
          tunnel: w465 -> [_ w488 w493 w498]
          tunnel: w461 -> [w483 w487 w489 w497]
          tunnel: [w483 w486 w492 w496] -> w449
          frame Default {
          }
          frame "Timing Control 1" {
            n173 = Variant To Data(type=0.0 ("Timing Control 1"), Variant=w488) -> (data=w485:dbl)  [unwired: 1 in, 1 out]
            n174 = Bundle By Name(cluster=w487, "Timing Control 1"=w485) -> (w486:T2)
          }
          frame "Timing Control 2" {
            n175 = Variant To Data(type=0.0 ("Timing Control 1"), Variant=w493) -> (data=w491:dbl)  [unwired: 1 in, 1 out]
            n176 = Bundle By Name(cluster=w489, "Timing Control 2"=w491) -> (w492:T2)
          }
          frame "Timing Control 3" {
            n177 = Variant To Data(type=0 ("Timing Control 1"), Variant=w498) -> (data=w495:i32)  [unwired: 1 in, 1 out]
            n178 = Bundle By Name(cluster=w497, "Timing Control 3"=w495) -> (w496:T2)
          }
        }
        n179 = Unbundle By Name(w449) -> ("Timing Mode"=w448:T7)
        n180 = call <vilib>:"svx_DAQ_SetTimingCaptions.vi"("Timing Mode (new)"=w448, "Timing Mode (old)"=w448, "Reference Cluster"=w453, "error in (no error)"=w454) -> ("Reference Cluster Out"=w452:T17, "error out"=w451:errorcluster)  [unwired: 7 in, 3 out]
        n181 = call <vilib>:"svx_DAQ_CheckChannelSettings.vi"("Display State In"=w449, "error in (no error)"=w451) -> ("Empty Channel List?"=w455:bool, "error out"=w456:errorcluster)  [unwired: 9 in, 3 out]
        n182 = case shown="False" w455 {
          tunnel: w460 -> [w475 w477]
          tunnel: [w474 w477] -> w459
          tunnel: w452 -> [w473 w479]
          tunnel: [w472 w478] -> w458
          tunnel: [w471 w481] -> w457
          tunnel: w449 -> [w470 w480]
          tunnel: w456 -> [w469 w482]
          tunnel: [TRUE ("Data Changed?") FALSE ("Data Changed?")] -> w450
          frame False {
            n183 = call <vilib>:"svx_DAQ_ConfigureTask.vi"("Task In"=w475, "Display State In"=w470, "cluster"=w473, "error in"=w469) -> ("task out"=w474:refnum<k21>, "Display State Out"=w472:T2, "error out"=w471:errorcluster)  [unwired: 8 in, 1 out]
          }
          frame True {
            n184 = call <vilib>:"svx_DAQ_ConfigureTiming.vi"("Display State In"=w480, "cluster"=w479, "Error In (no error)"=w482) -> ("Display State Out"=w478:T2, "error out"=w481:errorcluster)  [unwired: 9 in, 2 out]
          }
        }
        n185 = Bundle By Name(cluster=w464, "Data Changed?"=w450, "State Changed?"=TRUE) -> (w463:T1)
      }
      event "Channel Info Array": Value Change {
        w517 = TRUE ("Data Changed?")
        n186 = event-data() -> ("OldVal"=w509:T3[], "NewVal"=w508:T3[])  [unwired: 1 in]
        n187 = call <vilib>:"svx_DAQ_FindChannelChanges.vi"("New Value"=w508, "Old Value"=w509) -> ("Channel Array Out"=w514:T3[])  [unwired: 9 in]
        n188 = call <vilib>:"svx_DAQ_UpdateChannels.vi"("Channel Array In"=w514, "Display State In"=w510, "Reference Cluster"=w515, "error in (no error)"=w516) -> ("Display State Out"=w503:T2, "Reference Cluster Out"=w504:T17, "error out"=w507:errorcluster)  [unwired: 9 in]
        n189 = call <vilib>:"svx_DAQ_UpdateTachSection.vi"("State"=w503, "cluster"=w504, "error in (no error)"=w507) -> ("State Out"=w502:T2, "cluster"=w501:T17, "error out"=w505:errorcluster)  [unwired: 10 in]
        n190 = call <vilib>:"svx_DAQ_UpdateTriggerSection.vi"("State"=w502, "Reference Cluster"=w501, "error in (no error)"=w505) -> ("State Out"=w499:T2, "Reference Cluster Out"=w500:T17, "error out"=w506:errorcluster)  [unwired: 10 in]
        n191 = call <vilib>:"svx_DAQ_ConfigureTask.vi"("Task In"=w513, "Display State In"=w499, "cluster"=w500, "error in"=w506) -> ("task out"=w518:refnum<k21>, "Display State Out"=w511:T2, "error out"=w512:errorcluster)  [unwired: 8 in, 1 out]
        n192 = Bundle By Name(cluster=w519, "State Changed?"=w517, "Data Changed?"=w517) -> (w520:T1)
      }
      event Key Down? {
        w534 = refnum<vi> refnum  # Control
        # "This event adds key navigation features for quicker channel table editing during run time.\nTab should advance to next/right element in row, Shift Tab should move to previous/left element in row.\nReturn and Enter should advance to the same element in the next (channel) array element."
        n193 = event-data() -> ("VKey"=w527:T21, "Char"=w533:i16, "FocusObj"=w522:refnum<vi>, "PlatMods.Shift"=w523:bool)  [unwired: 1 in]
        n194 = property on="Channel Information" class="Clust (strict)"() -> ("Controls[]"=w525:refnum<vi>[])  [unwired: 2 in, 2 out]
        n195 = case shown="Default" w527 {
          tunnel: [w556 _] -> w531
          frame "Enter", "Return" {
            w556 = TRUE  # advance row
          }
          frame Default {
          }
        }
        n196 = case shown="\"ASCII\"" w527 {
          tunnel: w533 -> [w559 _]
          tunnel: [w557 _] -> w526
          frame "ASCII" {
            n197 = Equal?(x=w559, y=i16 9) -> (x = y?=w557:bool)
          }
          frame Default {
          }
        }
        n198 = To More Specific Class(target class=w534, reference=w522) -> (specific class reference=w524:refnum<vi>)  [unwired: 1 in, 1 out]
        n199 = Search 1D Array(1D array=w525, element=w524) -> (index of element=w521:i32)  [unwired: 1 in]
        n200 = case shown="1.." w521 {
          selector: w521 -> [_ w536]
          tunnel: w526 -> [_ w542]
          tunnel: w523 -> [_ w541]
          tunnel: w531 -> [_ w540]
          tunnel: w525 -> [_ w539]
          tunnel: [_ w537] -> w528
          frame Default {
            # "The key down wasn't with one of the channel table cells in focus"
          }
          frame 1.. {
            n201 = Or(x=w540, y=w542) -> (x .or. y?=w538:bool)
            n202 = case shown="True" w538 {
              selector: w538 -> [_ w552]
              tunnel: w541 -> [_ w554]
              tunnel: w539 -> [_ w553]
              tunnel: [_ w552] -> w537
              tunnel: w536 -> [_ w551]
              frame False {
                # "Not a recognized key combination for changing active cell."
              }
              frame True {
                # "Same row, move +/-1 cluster element"
                # "This case takes actions necessary to move focus. Discard LV event in favor of custom action implemented in this case."
                n203 = Decrement(x=w551) -> (x-1=w544:i32)
                n204 = Increment(x=w551) -> (x+1=w545:i32)
                n205 = Select(t=w544, s=w554, f=w545) -> (s? t:f=w543:i32)
                n206 = Array Size(array=w553) -> (size(s)=w555:i32)
                n207 = Quotient & Remainder(x=w543, y=w555) -> (x-y*floor(x/y)=w547:i32)  [unwired: 1 out]
                n208 = Max & Min(x=w547, y=1) -> (max(x,y)=w550:i32)  [unwired: 1 out]
                n209 = Index Array(array=w553, index=w550) -> (element=w549:refnum<vi>)
                n210 = property class="Ctl"(reference=w549, "Key Focus"=TRUE) -> ()  [unwired: 1 in, 2 out]
              }
            }
          }
        }
        n211 = event-data("Discard?"=w528) -> ()  [unwired: 1 in, 1 out]
      }
    }
  }
  "Display State Out" <- w32
  "Data Out" <- w28
  "Action" <- w31
